vi "pp3_updateSessionInfo.vi"(10 "Session info In":T1 {"T Jump%" format="%.3g"; "N Jump%" format="%.3g"; "G Jump%" format="%.3g"}, 11 "State In":T2={"Curr  tr"=0, "Curr (ms)"=0, "Cum (ms)"=0, "Run loop diff"=0, "Tone countdown (ms)"=0, "Countdown (ms)"=0, "Curr State"=enum."0 NULL", "Prev State"=enum."0 NULL", "Rw"=FALSE, "Sw"=FALSE, "Tone\nGate"=FALSE, "Punish"=FALSE, "Current DAQ DO Int"=0, "Current Loaded Trial"={"Trial Type Number"=1, "Trial Type"=enum."GO", "Trial Weight"=100, "Shock (mA)"=0.3, "Duration (ms)"=0.25, "Sound Type"=enum."04 FM Sweep", "Stim P1"=4000.0, "Stim P2"=0.0, "Stim P3"=0.0, "Stim P4"=2000.0, "DAQ Amplitude (V)"=0.25}, "Next Trial (for display purposes)"={"Trial Type Number"=1, "Trial Type"=enum."GO", "Trial Weight"=100, "Shock (mA)"=0.3, "Duration (ms)"=0.25, "Sound Type"=enum."04 FM Sweep", "Stim P1"=4000.0, "Stim P2"=0.0, "Stim P3"=0.0, "Stim P4"=2000.0, "DAQ Amplitude (V)"=0.25}, "Total trials memo"=0, "State start cum memo (ms)"=0, "Last dur jump time memo (ms)"=0, "Last dur shock time memo (ms)"=0, "Tone repeat memo (ms)"=0, "Webcam on"=FALSE, "Webcam recording"=FALSE, "State update flag"=FALSE, "Last loaded shock voltage"=0.0, "Vid upd"=enum."0"} {"Current DAQ DO Int" format="%016b"; "Next Trial (for display purposes)"."DAQ Amplitude (V)" min=0.0 max=5.0 format="%_6g"; "Next Trial (for display purposes)"."Shock (mA)" min=-1.0 max=5.0; "Next Trial (for display purposes)"."Trial Weight" step=1; "Next Trial (for display purposes)"."Duration (ms)" min=0.0 max=1.0; "Next Trial (for display purposes)"."Trial Type Number" min=1 max=256 step=1; "Current Loaded Trial"."DAQ Amplitude (V)" min=0.0 max=5.0 format="%_6g"; "Current Loaded Trial"."Shock (mA)" min=-1.0 max=5.0; "Current Loaded Trial"."Trial Weight" step=1; "Current Loaded Trial"."Duration (ms)" min=0.0 max=1.0; "Current Loaded Trial"."Trial Type Number" min=1 max=256 step=1}) -> (2 "Session info Out":T1 {"T Jump%" format="%.3g"; "N Jump%" format="%.3g"; "G Jump%" format="%.3g"})   [LabVIEW 2013]
uses:
  pp3_CTL_StateInfo.ctl
  pp2_CTL_State.ctl
  pp3_CTL_Trial.ctl
  pp3_CTL_TrialType.ctl
  labolabo2/waveforms/WFTypes.ctl
  pp3_CTL_SessionInfo.ctl
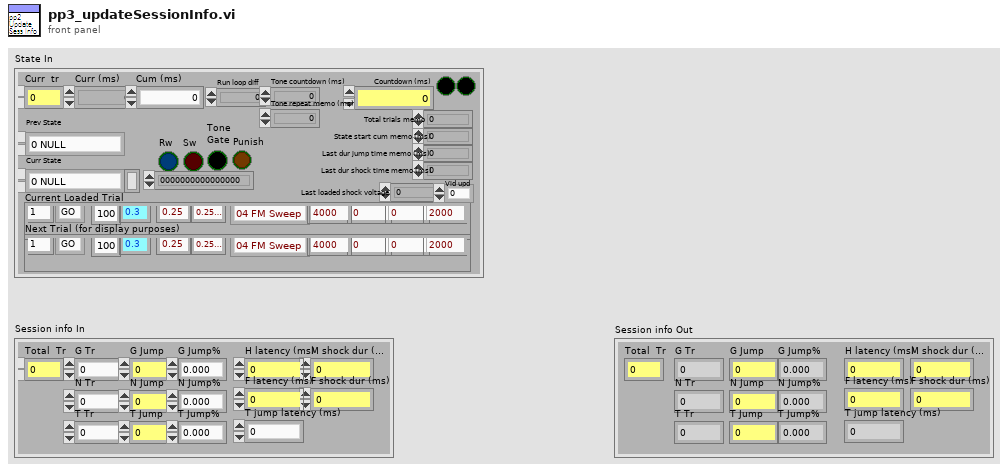
[diagram p1: front panel]
types:
  T1 = typedef "pp3_CTL_SessionInfo.ctl" = cluster{"Total  Tr":u32, "G Tr":u32, "G Jump":u32, "G Jump%":dbl, "N Tr":u32, "N Jump":u32, "N Jump%":dbl, "T Tr":u32, "T Jump":u32, "T Jump%":dbl, "M shock dur (ms)":dbl, "F shock dur (ms)":dbl, "H latency (ms)":dbl, "F latency (ms)":dbl, "T jump latency (ms)":dbl}
  T2 = typedef "pp3_CTL_StateInfo.ctl" = cluster{"Curr  tr":u16, "Curr (ms)":u32, "Cum (ms)":i64, "Run loop diff":i64, "Tone countdown (ms)":i64, "Countdown (ms)":i64, "Curr State":T3, "Prev State":T3, "Rw":bool, "Sw":bool, "Tone\nGate":bool, "Punish":bool, "Current DAQ DO Int":u16, "Current Loaded Trial":T4, "Next Trial (for display purposes)":T4, "Total trials memo":i64, "State start cum memo (ms)":i64, "Last dur jump time memo (ms)":i64, "Last dur shock time memo (ms)":i64, "Tone repeat memo (ms)":i64, "Webcam on":bool, "Webcam recording":bool, "State update flag":bool, "Last loaded shock voltage":dbl, "Vid upd":enum16{"0", "1", "2", "3", "4", "5", "6", "7", "8", "9"}}
  T3 = typedef "pp2_CTL_State.ctl" = enum8{"0 NULL", "1 Habituation", "2 (Load Trial)", "3 Stay Period", "4 Load Audio/Click Delay", "5 GO Trial", "6 GO Jumped", "7 GO Timeout", "8 NOGO Trial", "9 NOGO Jumped", "10 NOGO Timeout", "11 TEST Trial", "12 TEST Jumped", "13 TEST Timeout", "14 Intertrial Interval", "15 Done"}
  T4 = typedef "pp3_CTL_Trial.ctl" = cluster{"Trial Type Number":i16, "Trial Type":T5, "Trial Weight":u32, "Shock (mA)":dbl, "Duration (ms)":dbl, "Sound Type":T6, "Stim P1":dbl, "Stim P2":dbl, "Stim P3":dbl, "Stim P4":dbl, "DAQ Amplitude (V)":dbl}
  T5 = typedef "pp3_CTL_TrialType.ctl" = enum16{"OFF", "GO", "NOGO", "TEST"}
  T6 = typedef "WFTypes.ctl" = enum16{"00 NULL", "01 DC", "02 Noise", "03 Pure Tone", "04 FM Sweep"}
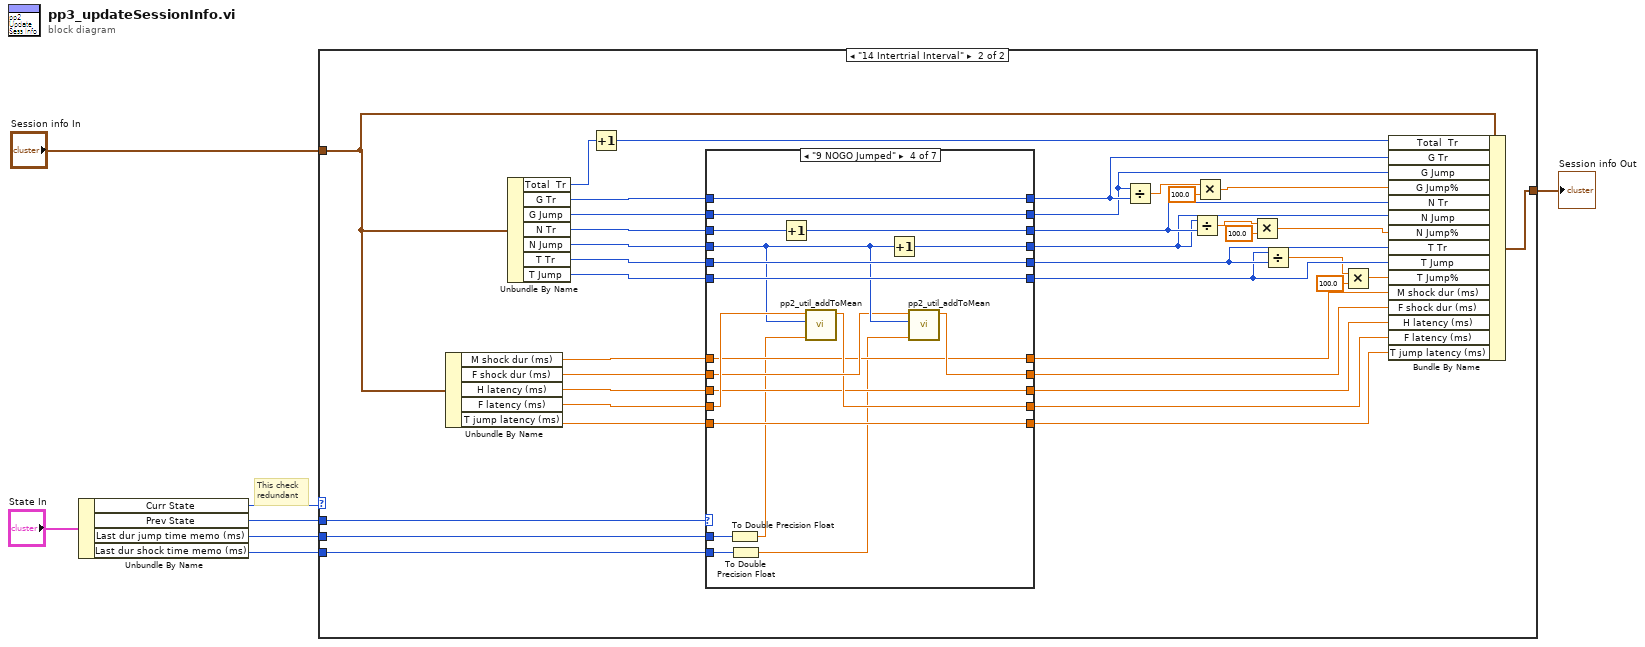
[diagram p0: block diagram]
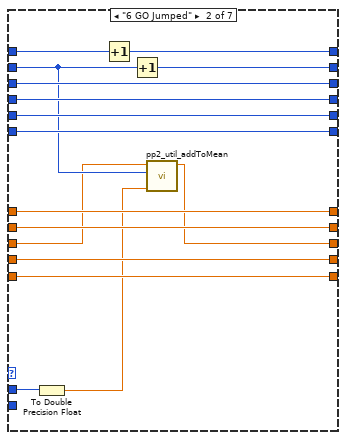
[diagram p4: hidden frame]
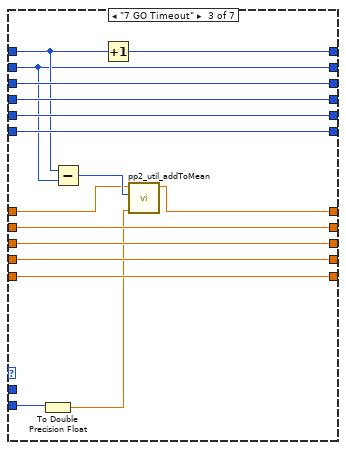
[diagram p5: hidden frame]
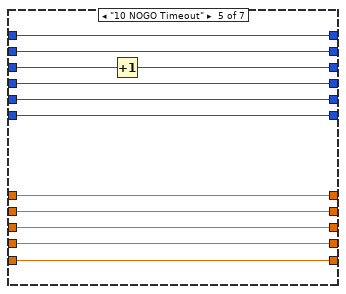
[diagram p6: hidden frame]
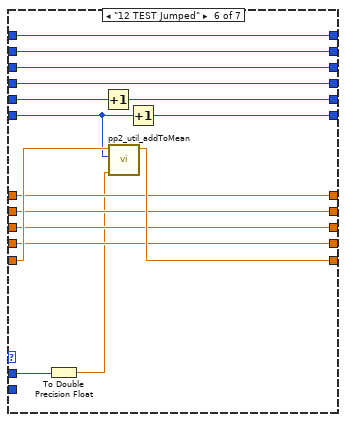
[diagram p7: hidden frame]
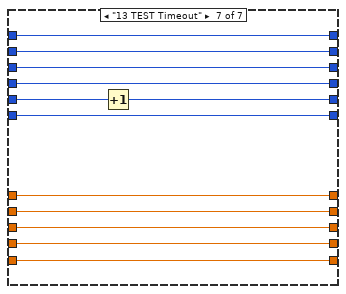
[diagram p8: hidden frame]
diagram:
  # "This check\nredundant"
  n1 = Unbundle By Name("State In") -> ("Curr State"=w1:T3, "Prev State"=w6:T3, "Last dur jump time memo (ms)"=w4:i64, "Last dur shock time memo (ms)"=w3:i64)
  n2 = case shown="\"14 Intertrial Interval\"" w1 {
    tunnel: w6 -> [_ w32]
    tunnel: [w8 w31] -> w5
    tunnel: w4 -> [_ w30]
    tunnel: w3 -> [_ w29]
    tunnel: "Session info In" -> [w8 w23]
    frame Default {
    }
    frame "14 Intertrial Interval" {
      n3 = Unbundle By Name(w23) -> ("M shock dur (ms)"=w22:dbl, "F shock dur (ms)"=w18:dbl, "H latency (ms)"=w19:dbl, "F latency (ms)"=w20:dbl, "T jump latency (ms)"=w21:dbl)
      n4 = Unbundle By Name(w23) -> ("Total  Tr"=w46:u32, "G Tr"=w44:u32, "G Jump"=w43:u32, "N Tr"=w42:u32, "N Jump"=w41:u32, "T Tr"=w40:u32, "T Jump"=w39:u32)
      n5 = Increment(x=w46) -> (x+1=w45:u32)
      n6 = case shown="\"9 NOGO Jumped\"" w32 {
        tunnel: w44 -> [w57 w69 w84 w104 w117 w135 w147]
        tunnel: w43 -> [w56 w62 w83 w105 w118 w136 w148]
        tunnel: w42 -> [w55 w73 w88 w107 w120 w133 w145]
        tunnel: w41 -> [w54 w72 w87 w100 w114 w134 w146]
        tunnel: w40 -> [w53 w71 w86 w103 w116 w132 w144]
        tunnel: w39 -> [w52 w70 w85 w102 w115 w128 w142]
        tunnel: [w55 w73 w88 w106 w119 w133 w145] -> w36
        tunnel: [w54 w72 w87 w108 w114 w134 w146] -> w35
        tunnel: [w53 w71 w86 w103 w116 w131 w143] -> w34
        tunnel: [w52 w70 w85 w102 w115 w130 w142] -> w33
        tunnel: [w57 w68 w89 w104 w117 w135 w147] -> w38
        tunnel: [w56 w63 w83 w105 w118 w136 w148] -> w37
        tunnel: w22 -> [w51 w67 w77 w94 w113 w126 w141]
        tunnel: w18 -> [w50 w66 w79 w99 w112 w125 w140]
        tunnel: w19 -> [w47 w61 w82 w95 w111 w124 w139]
        tunnel: w20 -> [w48 w65 w81 w101 w110 w123 w138]
        tunnel: w21 -> [w49 w64 w80 w96 w109 w129 w137]
        tunnel: w30 -> [_ w59 _ w93 _ w122 _]
        tunnel: w29 -> [_ _ w75 w92 _ _ _]
        tunnel: [w51 w67 w76 w94 w113 w126 w141] -> w28
        tunnel: [w50 w66 w79 w98 w112 w125 w140] -> w27
        tunnel: [w49 w64 w80 w96 w109 w127 w137] -> w24
        tunnel: [w48 w65 w81 w97 w110 w123 w138] -> w25
        tunnel: [w47 w60 w82 w95 w111 w124 w139] -> w26
        frame Default {
        }
        frame "6 GO Jumped" {
          n7 = To Double Precision Float(number=w59) -> (double precision float=w58:dbl)
          n8 = Increment(x=w69) -> (x+1=w68:u32)
          n9 = Increment(x=w62) -> (x+1=w63:u32)
          n10 = call "pp2_util_addToMean.vi"("New value"=w58, "Original count"=w62, "Original mean"=w61) -> ("New mean"=w60:dbl)  [unwired: 8 in]
        }
        frame "7 GO Timeout" {
          n11 = To Double Precision Float(number=w75) -> (double precision float=w74:dbl)
          n12 = Subtract(x=w84, y=w83) -> (x-y=w78:u32)
          n13 = Increment(x=w84) -> (x+1=w89:u32)
          n14 = call "pp2_util_addToMean.vi"("New value"=w74, "Original count"=w78, "Original mean"=w77) -> ("New mean"=w76:dbl)  [unwired: 8 in]
        }
        frame "9 NOGO Jumped" {
          n15 = To Double Precision Float(number=w93) -> (double precision float=w91:dbl)
          n16 = To Double Precision Float(number=w92) -> (double precision float=w90:dbl)
          n17 = Increment(x=w107) -> (x+1=w106:u32)
          n18 = call "pp2_util_addToMean.vi"("New value"=w91, "Original count"=w100, "Original mean"=w101) -> ("New mean"=w97:dbl)  [unwired: 8 in]
          n19 = Increment(x=w100) -> (x+1=w108:u32)
          n20 = call "pp2_util_addToMean.vi"("New value"=w90, "Original count"=w100, "Original mean"=w99) -> ("New mean"=w98:dbl)  [unwired: 8 in]
        }
        frame "10 NOGO Timeout" {
          n21 = Increment(x=w120) -> (x+1=w119:u32)
        }
        frame "12 TEST Jumped" {
          n22 = To Double Precision Float(number=w122) -> (double precision float=w121:dbl)
          n23 = Increment(x=w132) -> (x+1=w131:u32)
          n24 = call "pp2_util_addToMean.vi"("New value"=w121, "Original count"=w128, "Original mean"=w129) -> ("New mean"=w127:dbl)  [unwired: 8 in]
          n25 = Increment(x=w128) -> (x+1=w130:u32)
        }
        frame "13 TEST Timeout" {
          n26 = Increment(x=w144) -> (x+1=w143:u32)
        }
      }
      n27 = Divide(x=w37, y=w38) -> (x/y=w17:dbl)
      n28 = Divide(x=w35, y=w36) -> (x/y=w10:dbl)
      n29 = Multiply(x=w17, y=100.0) -> (x*y=w11:dbl)
      n30 = Multiply(x=w10, y=100.0) -> (x*y=w12:dbl)
      n31 = Divide(x=w33, y=w34) -> (x/y=w9:dbl)
      n32 = Multiply(x=w9, y=100.0) -> (x*y=w13:dbl)
      n33 = Bundle By Name(cluster=w23, "Total  Tr"=w45, "G Tr"=w38, "G Jump"=w37, "G Jump%"=w11, "N Tr"=w36, "N Jump"=w35, "N Jump%"=w12, "T Tr"=w34, "T Jump"=w33, "T Jump%"=w13, "M shock dur (ms)"=w28, "F shock dur (ms)"=w27, "H latency (ms)"=w26, "F latency (ms)"=w25, "T jump latency (ms)"=w24) -> (w31:T1)
    }
  }
  "Session info Out" <- w5
